vi "Solve Linear Equations By LU.vi"(3 "Known Vector":dbl[](array[numeric]) format="%.2f", 4 "Input Matrix":T1) -> (0 "error":i32, 1 "Solution Vector":dbl[](array[numeric]) format="%.2f")   [LabVIEW 2010, in "NI_AALBase.lvlib"]
doc: "Solves a real linear system AX=Y using LU factorization."
uses:
  NI_AALBase.lvlib
  RealMatrix.ctl
  lvanlys.dll
  NI_Matrix.lvlib
panel:
  # "Solve General Linear Equations"
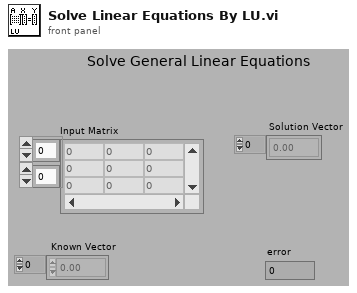
[diagram p1: front panel]
types:
  T1 = typedef "NI_Matrix.lvlib/RealMatrix.ctl" = dbl[][]
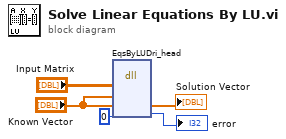
[diagram p0: block diagram]
diagram:
  n1 = dll-call lib="C:/Program Files/National Instruments/LabVIEW 2010/resource/lvanlys.*" fn="EqsByLUDri_head"("Input Matrix"="Input Matrix", "Known Vector"="Known Vector", "Known Vector"="Known Vector", 0) -> ("Known Vector"=→"Solution Vector":dbl[], →"error":i32)  [unwired: 6 in, 2 out]
